vi "条件结构-平方根.vi"() -> ()   [LabVIEW 2015]
panel:
  out "输入":dbl
  in  "请输入n":dbl
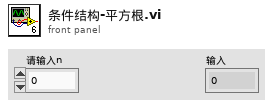
[diagram p1: front panel]
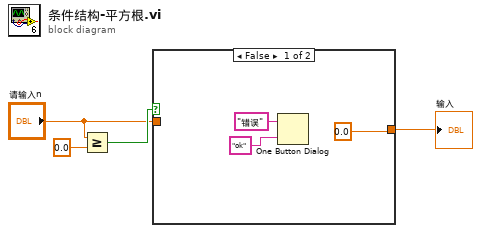
[diagram p0: block diagram]
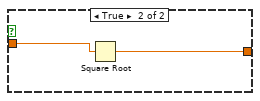
[diagram p2: hidden frame]
diagram:
  n1 = Greater Or Equal?(x="请输入n", y=0.0) -> (x >= y?=w3:bool)
  n2 = case shown="False" w3 {
    tunnel: "请输入n" -> [_ w9]
    tunnel: [0.0 w8] -> w1
    frame False {
      n3 = One Button Dialog(message="错误", button name ("OK")="ok") -> ()  [unwired: 1 out]
    }
    frame True {
      n4 = Square Root(x=w9) -> (sqrt(x)=w8:dbl)
    }
  }
  "输入" <- w1
